vi "Loading option.vi"() -> (3 "options":i32)   [LabVIEW 2021, in "Migrator Reusables.lvlib"]
uses:
  Migrator Reusables.lvlib
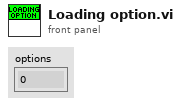
[diagram p1: front panel]
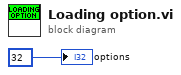
[diagram p0: block diagram]
diagram:
  "options" <- 32 ("options")
